vi "Periodic Tasks.vi"(8 "error in":errorcluster) -> ()   [LabVIEW 2015]
doc: "This VI runs in parallel to other tasks. It can contain as many user-defined periodic loops as you need. These can carry out PID or other sorts of timed response."
uses:
  <vilib>/Rock Robotics/WPI/Utilities/WPI_GetSetVariantRefNum.vi
  ADI MXP IMU/ADI MXP IMU/FRC ADI MXP IMU.lvlib
panel:
  in  "Angle":dbl=90.0 format="%#_13g"
  in  "Spin Speed":dbl=0.5
  in  "Button":i32=7
  in  "Bouton":i32
  in  "Push Angle":i16=170 min=0 max=170 step=1
  in  "Action Time":u32=700
  # "Poussoir"
  # "(ms)"
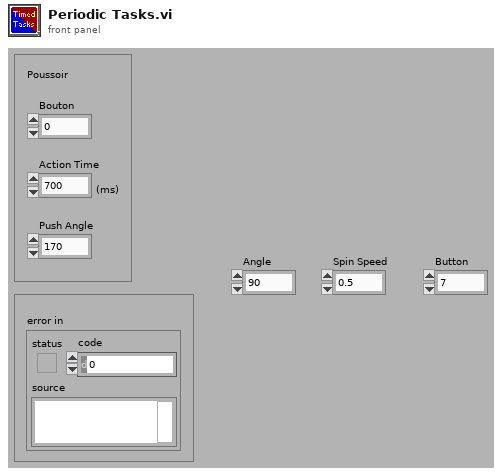
[diagram p1: front panel]
types:
  T1 = typedef "WPI_RobotDriveDevRef.ctl" = cluster{"DevStatus":errorcluster, "Motors[]":T2[], "Square Inputs":bool, "Max Output":dbl}
  T2 = typedef "WPI_MotorControlDeviceRef.ctl" = cluster{"DeviceStatus":errorcluster, "Type":T3, "PWM":cluster{"PWM Channel":T4, "DeadBand":T5}, "CAN":cluster{"Device Number":u8, "Control Mode":T6, "Semaphore":T7, "Max Vout":dbl, "TalonSRX Control Mode":T8}, "Invert":bool}
  T3 = typedef "WPI_MotorControlType.ctl" = enum16{"PWM", "CAN", "CANTalonSRX"}
  T4 = typedef "FPGA_DIOPWMChannel.ctl" = enum8{"PWM 0", "PWM 1", "PWM 2", "PWM 3", "PWM 4", "PWM 5", "PWM 6", "PWM 7", "PWM 8", "PWM 9", "PWM MXP 0", "PWM MXP 1", "PWM MXP 2", "PWM MXP 3", "PWM MXP 4", "PWM MXP 5", "PWM MXP 6", "PWM MXP 7", "PWM MXP 8", "PWM MXP 9", "Invalid"}
  T5 = typedef "WPI_PWMDeadband.ctl" = cluster{"Name":string, "maxPositivePwm":i32, "minPositivePwm":i32, "centerPwm":i32, "maxNegativePwm":i32, "minNegativePwm":i32, "angularRange":u16}
  T6 = typedef "WPI_CANJaguar_ControlMode.ctl" = enum8{"Percent VBus", "Current", "Speed", "Position", "Voltage"}
  T7 = typedef "Semaphore RefNum" = refnum<k1>
  T8 = typedef "WPI_CANTalonSRX_APIControlMode.ctl" = enum8{"Percent VBus", "Speed", "Position", "Slave", "Unchanged / Invalid", "Voltage Compensation", "Current", "Motion Profile"}
  T9 = typedef "FRC ADI MXP IMU.lvlib/WPI_AnalogDevicesIMUInterruptDevRef.ctl" = cluster{"SimpleGyroDevRef":T10, "InterruptRef":T12}
  T10 = typedef "FRC ADI MXP IMU.lvlib/WPI_AnalogDevicesIMUDevRef.ctl" = cluster{"DevStatus":errorcluster, "Handle":i32, "SPI Bus":T11, "Device Found":bool, "Sample Rate":dbl, "Device Ready":bool, "Yaw Axis":enum16{"X", "Y", "Z"}, "AHRS Algorithm":enum16{"Complementary", "Madgwick"}}
  T11 = typedef "spi_bus.ctl" = enum16{"SPI On-Board, CS0", "SPI On-Board, CS1", "SPI On-Board, CS2", "SPI On-Board, CS3", "SPI MXP", "Invalid"}
  T12 = typedef "WPI_InterruptRef.ctl" = cluster{"DevStatus":errorcluster, "InterruptIndex":T13}
  T13 = typedef "FPGA_InterruptIndex.ctl" = enum8{"0", "1", "2", "3", "4", "5", "6", "7", "Invalid"}
  T14 = typedef "WPI_ServoDeviceRef.ctl" = cluster{"DeviceStatus":errorcluster, "PWM Channel":T4, "DeadBand":T5}
  T15 = typedef "WPI_JoystickDevRef.ctl" = cluster{"Device":T16}
  T16 = typedef "WPI_JoystickDeviceEnum.ctl" = enum16{"USB 0", "USB 1", "USB 2", "USB 3", "USB 4", "USB 5"}
  T17 = cluster{"ServoDeviceRef":T14, "JoystickDevRef":T15, "JoystickDevRef":T15}
  T18 = cluster{"X Angle":dbl, "Y Angle":dbl, "Z Angle":dbl}
  T19 = typedef "WPI_SwitchDevRef.ctl" = cluster{"DevStatus":errorcluster, "DIO Channel":T20, "CntIndex":T21, "Normally Closed":bool}
  T20 = typedef "FPGA_DIOChannel.ctl" = enum8{"DIO 0", "DIO 1", "DIO 2", "DIO 3", "DIO 4", "DIO 5", "DIO 6", "DIO 7", "DIO 8", "DIO 9", "DIO MXP 0", "DIO MXP 1", "DIO MXP 2", "DIO MXP 3", "DIO MXP 4", "DIO MXP 5", "DIO MXP 6", "DIO MXP 7", "DIO MXP 8", "DIO MXP 9", "DIO MXP 10", "DIO MXP 11", "DIO MXP 12", "DIO MXP 13", "DIO MXP 14", "DIO MXP 15", "Invalid"}
  T21 = typedef "FPGA_CounterCtrSystemIndex.ctl" = enum8{"Ctr 0", "Ctr 1", "Ctr 2", "Ctr 3", "Ctr 4", "Ctr 5", "Ctr 6", "Ctr 7", "Invalid"}
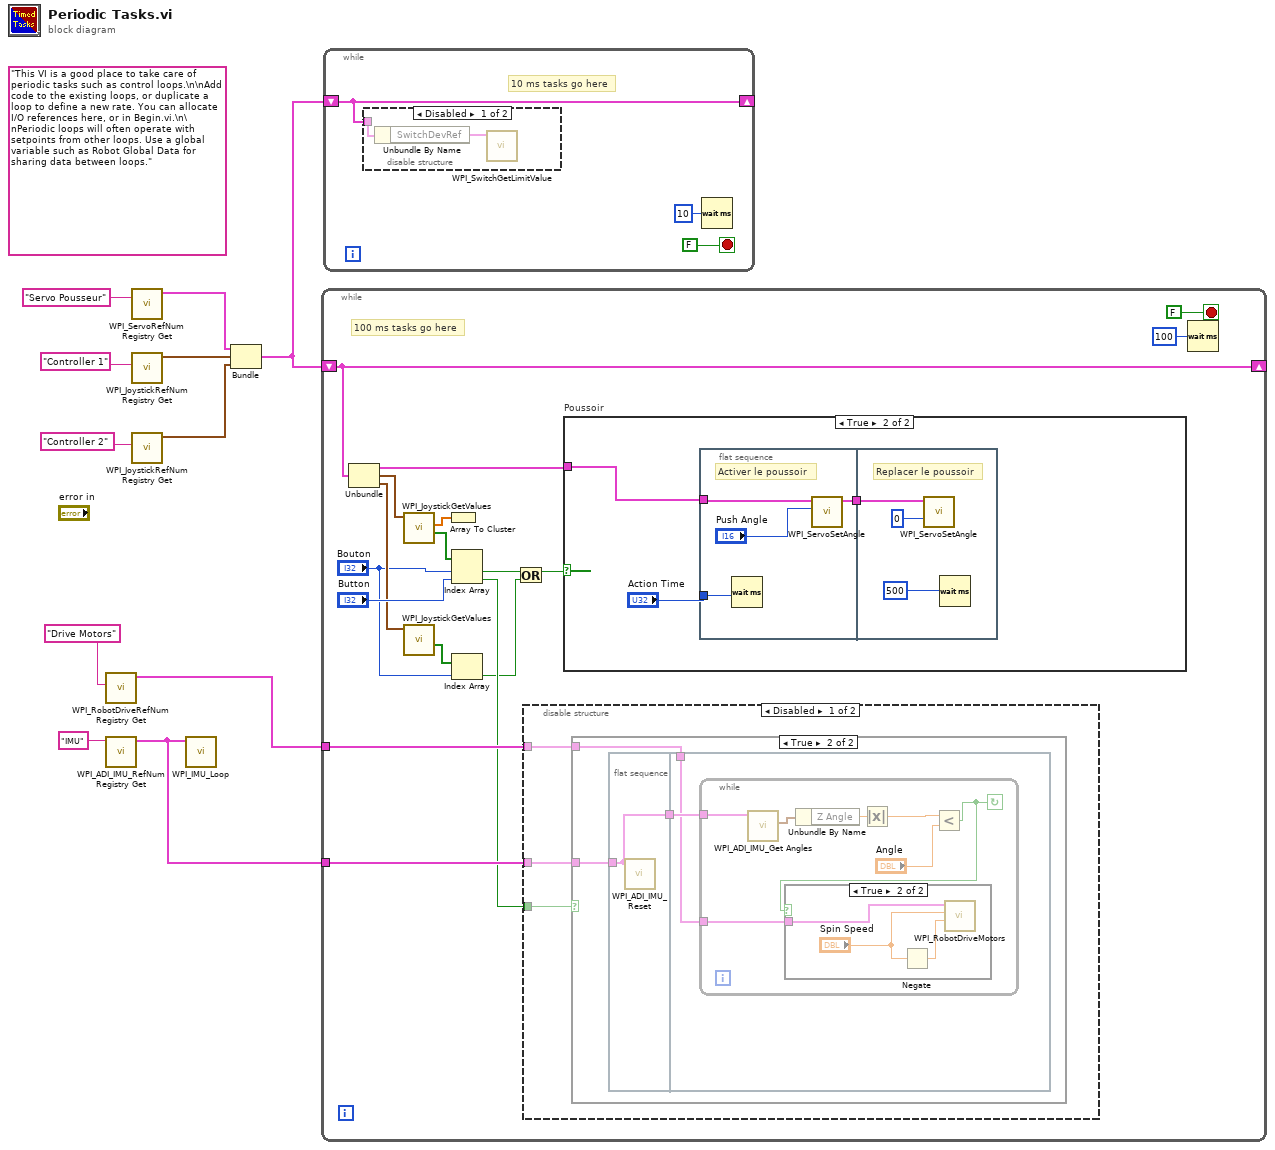
[diagram p0: block diagram]
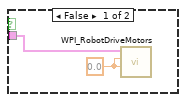
[diagram p3: hidden frame]
diagram:
  (unwired) "This VI is a good place to take care of periodic tasks such as control loops.\n\nAdd code to the existing loops, or duplicate a loop to define a new rate. You can allocate I/O references here, or in Begin.vi.\n\nPeriodic loops will often operate with setpoints from other loops. Use a global variable such as Robot Global Data for sharing data between loops."
  n1 = call <vilib>:"WPI_RobotDriveRefNum Registry Get.vi"("refnum name"="Drive Motors") -> ("RobotDriveDevRef"=w3:T1)  [unwired: 9 in, 1 out]
  n2 = call "WPI_ADI_IMU_RefNum Registry Get.vi"("refnum name"="IMU") -> ("ADI IMU Interrupt DevRef"=w5:T9)  [unwired: 9 in, 1 out]
  n3 = call <vilib>:"WPI_ServoRefNum Registry Get.vi"("refnum name"="Servo Pousseur") -> ("ServoDeviceRef"=w8:T14)  [unwired: 9 in, 1 out]
  n4 = call <vilib>:"WPI_JoystickRefNum Registry Get.vi"("refnum name"="Controller 1") -> ("JoystickDevRef"=w7:T15)  [unwired: 1 in, 9 out]
  n5 = call <vilib>:"WPI_JoystickRefNum Registry Get.vi"("refnum name"="Controller 2") -> ("JoystickDevRef"=w1:T15)  [unwired: 1 in, 9 out]
  n6 = call "WPI_IMU_Loop.vi"("ADI IMU Interrupt DevRef"=w5) -> ()  [unwired: 10 in, 1 out]
  n7 = Bundle("ServoDeviceRef"=w8, "JoystickDevRef"=w7, "JoystickDevRef"=w1) -> (w10:T17)  [unwired: 1 out]
  n8 = while {
    shift-right: [w26] -> _
    shift-left: w10 -> [w26]
    tunnel: w5 -> [w20]
    tunnel: w3 -> [w19]
    stop <- FALSE stop-if-true
    # "100 ms tasks go here"
    n9 = Unbundle(w26) -> ("ServoDeviceRef"=w25:T14, "JoystickDevRef"=w24:T15, "JoystickDevRef"=w16:T15)
    n10 = call <vilib>:"WPI_JoystickGetValues.vi"("JoystickDevRef"=w24) -> ("Buttons"=w23:bool[], "Axes"=w22:dbl[])  [unwired: 6 in, 3 out]
    n11 = call <vilib>:"WPI_JoystickGetValues.vi"("JoystickDevRef"=w16) -> ("Buttons"=w15:bool[])  [unwired: 6 in, 4 out]
    n12 = Array To Cluster(array=w22) -> ()  [unwired: 1 out]
    n13 = Index Array(array=w23, index #1="Bouton", index #2="Button") -> (element #1=w17:bool, element #2=w18:bool)
    n14 = Index Array(array=w15, index="Bouton") -> (element=w12:bool)
    n15 = Or(x=w17, y=w12) -> (x .or. y?=w14:bool)
    n16 = disable-structure "Diagram Disable Structure" shown="Disabled" {
      disable-tunnel: w20 -> [w31 _]
      disable-tunnel: w19 -> [w30 _]
      disable-tunnel: w18 -> [w29 _]
      frame Disabled {
        n17 = case shown="True" w29 {
          tunnel: w31 -> [_ w33]
          tunnel: w30 -> [_ w32]
          frame False {
          }
          frame True {
            n18 = flat-sequence {
              tunnel: w33 -> [w35]
              tunnel: [w35] -> w34
              tunnel: w34 -> [w37]
              tunnel: w32 -> [w36]
              frame #0 {
                n19 = call "WPI_ADI_IMU_Reset.vi"("ADI IMU Interrupt DevRef"=w35) -> ()  [unwired: 9 in, 2 out]
              }
              frame #1 {
                n20 = while {
                  tunnel: w37 -> [w40]
                  tunnel: w36 -> [w38]
                  stop <- w39 continue-if-true
                  n21 = call "WPI_ADI_IMU_Get Angles.vi"("ADI IMU Interrupt DevRef"=w40) -> ("IMU Angles"=w44:T18)  [unwired: 7 in, 3 out]
                  n22 = Unbundle By Name(w44) -> ("Z Angle"=w43:dbl)
                  n23 = Absolute Value(x=w43) -> (abs(x)=w41:dbl)
                  n24 = Less?(x=w41, y="Angle") -> (x < y?=w39:bool)
                  n25 = case shown="True" w39 {
                    tunnel: w38 -> [w45 w47]
                    frame False {
                      w46 = 0.0 ("RightSpeed")
                      n26 = call <vilib>:"WPI_RobotDriveMotors.vi"("RightSpeed"=w46, "LeftSpeed"=w46, "RobotDriveDevRef"=w45) -> ()  [unwired: 6 in, 3 out]
                    }
                    frame True {
                      n27 = Negate(x="Spin Speed") -> (-x=w49:dbl)
                      n28 = call <vilib>:"WPI_RobotDriveMotors.vi"("RightSpeed"=w49, "LeftSpeed"="Spin Speed", "RobotDriveDevRef"=w47) -> ()  [unwired: 6 in, 3 out]
                    }
                  }
                }
              }
            }
          }
        }
      }
      frame Enabled {
      }
    }
    n29 = case "Poussoir" shown="True" w14 {
      tunnel: w25 -> [_ w50]
      frame False {
      }
      frame True {
        n30 = flat-sequence {
          tunnel: [w56] -> w52
          tunnel: "Action Time" -> [w53]
          tunnel: w50 -> [w54]
          tunnel: w52 -> [w59]
          frame #0 {
            # "Activer le poussoir"
            n31 = Wait (ms)(milliseconds to wait=w53) -> ()  [unwired: 1 out]
            n32 = call <vilib>:"WPI_ServoSetAngle.vi"("Angle"="Push Angle", "ServoDeviceRef"=w54) -> ("ServoDeviceRef"=w56:T14)  [unwired: 8 in, 1 out]
          }
          frame #1 {
            # "Replacer le poussoir"
            n33 = call <vilib>:"WPI_ServoSetAngle.vi"("Angle"=0, "ServoDeviceRef"=w59) -> ()  [unwired: 8 in, 2 out]
            n34 = Wait (ms)(milliseconds to wait=u32 500) -> ()  [unwired: 1 out]
          }
        }
      }
    }
    n35 = Wait (ms)(milliseconds to wait=u32 100) -> ()  [unwired: 1 out]
  }
  n36 = while {
    shift-right: [w60] -> _
    shift-left: w10 -> [w60]
    stop <- FALSE stop-if-true
    # "10 ms tasks go here"
    n37 = disable-structure shown="Disabled" {
      disable-tunnel: w60 -> [w64 _]
      frame Disabled {
        n38 = Unbundle By Name(w64) -> ("SwitchDevRef"=w63:T19)
        n39 = call <vilib>:"WPI_SwitchGetLimitValue.vi"("SwitchDevRef"=w63) -> ()  [unwired: 8 in, 3 out]
      }
      frame Enabled {
      }
    }
    n40 = Wait (ms)(milliseconds to wait=u32 10) -> ()  [unwired: 1 out]
  }
